vi "Create.vi"(8 "error in (no error)":errorcluster, 10 "Channel":i8, 11 "TecellaClient.lvclass":refnum<class "TecellaClient.lvclass">) -> (0 "error out":errorcluster, 3 "TecellaChannel out":refnum<class "TecellaChannel.lvclass">)   [LabVIEW 2009, in "TecellaChannel.lvclass"]
uses:
  TecellaChannel.lvclass
  TecellaClient/TecellaClient.lvclass
  TecellaChannel.lvclass/TecellaChannel.ctl
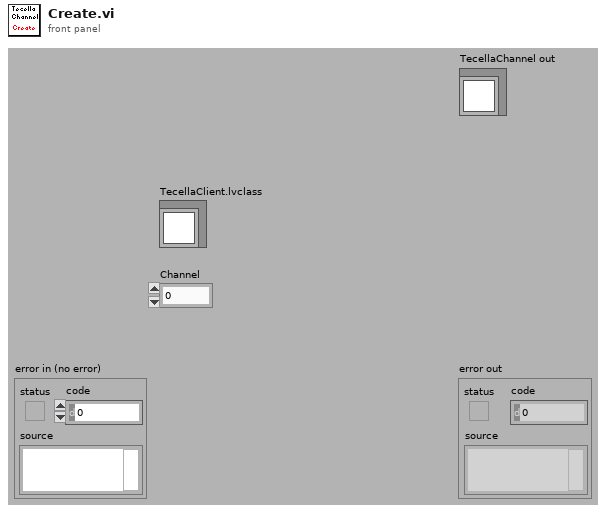
[diagram p1: front panel]
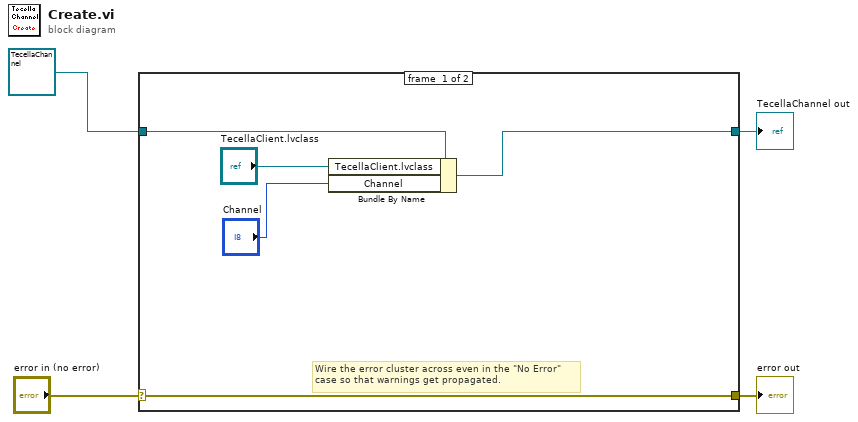
[diagram p0: block diagram]
diagram:
  n1 = case shown="No Error" "error in (no error)" {
    selector: "error in (no error)" -> [w9 w11]
    tunnel: [w9 w11] -> w3
    tunnel: [w7 w10] -> w1
    tunnel: refnum<class "TecellaChannel.lvclass"> refnum ("TecellaChannel in") -> [w8 w10]
    frame #0 {
      # "Wire the error cluster across even in the \"No Error\"\ncase so that warnings get propagated."
      n2 = Bundle By Name(cluster=w8, "TecellaClient.lvclass"="TecellaClient.lvclass", "Channel"="Channel") -> (w7:refnum<class "TecellaChannel.lvclass">)
    }
    frame #1 {
    }
  }
  "error out" <- w3
  "TecellaChannel out" <- w1
